vi "SendCallbackMsg.vi"(8 "error in (no error)":errorcluster, 10 "UpstreamMsg":refnum<class "UpstreamMsgParent.lvclass">, 11 "DownStreamMsgHandler in":refnum<class "DownStreamMsgHandler.lvclass">) -> (0 "error out":errorcluster, 3 "DownStreamMsgHandler out":refnum<class "DownStreamMsgHandler.lvclass">)   [LabVIEW 2020, in "DownstreamMsgHandler.lvlib" / "DownStreamMsgHandler.lvclass"]
uses:
  DownStreamMsgHandler.lvclass
  C:/Program Files (x86)/National Instruments/LabVIEW 2020/vi.lib/ActorFramework/Actor/Actor.lvclass
  UpstreamMsg/UpstreamMsgParent/UpstreamMsgParent.lvclass
  <vilib>/ActorFramework/Actor/Actor.lvclass/Actor.ctl
  ServiceManager Messages/SendUpstreamMessage Msg/SendUpstreamMessage Msg.lvclass/SendUpstreamMessage Msg.ctl
  <vilib>/ActorFramework/Message Enqueuer/Message Enqueuer.lvclass/Message Enqueuer.ctl
  <vilib>/ActorFramework/Message Enqueuer/Enqueue.vi
  ServiceManager Messages/SendUpstreamMessage Msg/SendUpstreamMessage Msg.lvclass
  C:/Program Files (x86)/National Instruments/LabVIEW 2020/vi.lib/ActorFramework/Message/Message.lvclass
  <vilib>/ActorFramework/Message Priority Queue/Priority Enqueue.vi
  <vilib>/ActorFramework/Actor/Actor.lvclass
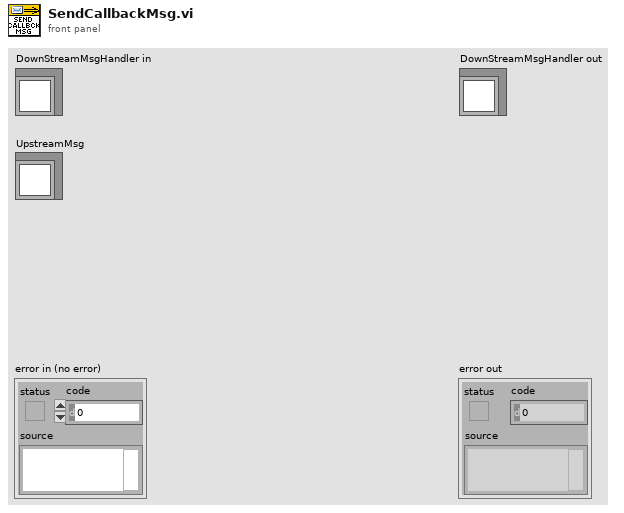
[diagram p1: front panel]
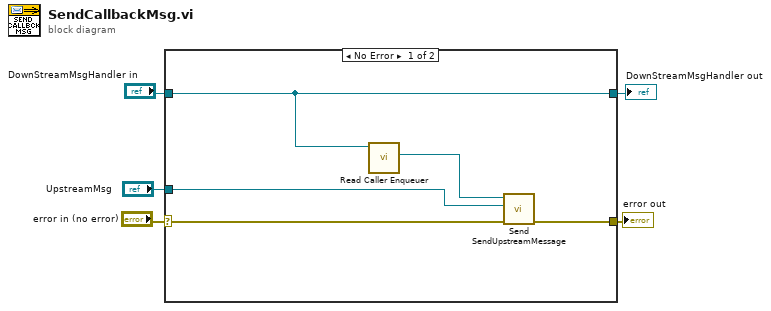
[diagram p0: block diagram]
diagram:
  n1 = case shown="No Error" "error in (no error)" {
    selector: "error in (no error)" -> [w7 w12]
    tunnel: [w6 w12] -> w4
    tunnel: [w10 w11] -> w2
    tunnel: "DownStreamMsgHandler in" -> [w10 w11]
    tunnel: "UpstreamMsg" -> [w8 _]
    frame No Error {
      n2 = call <vilib>:"Read Caller Enqueuer.vi"("Actor"=w10) -> ("Caller Enqueuer"=w9:refnum<class "Message Enqueuer.lvclass">)  [unwired: 10 in]
      n3 = call "Send SendUpstreamMessage.vi"("error in (no error)"=w7, "UpstreamMsg"=w8, "Message Enqueuer"=w9) -> ("error out"=w6:errorcluster)  [unwired: 7 in, 1 out]
    }
    frame Error {
    }
  }
  "error out" <- w4
  "DownStreamMsgHandler out" <- w2
